vi "read data.vi"(8 "error in (no error)":errorcluster, 9 "pDMAStatus":i32[](array[numeric]), 10 "Buffer":u16[](array[numeric]), 11 "task":T1={"Task Info"={"Accele Task"=[], "Simulate"=FALSE, "采样率"={"AISampleRate"=10123, "CouplingType"=10000, "Butter"=1000}, "Trig"={"PreTrigCNT"=0, "TriggerMode"=enum."中间触发", "TriggerSource"=enum."软件触发", "ATRTriggerChannel"=enum."通道0", "TriggerDir"=enum."下降沿触发", "TrigLevelVolt"=0.0, "bAvailableTrig"=FALSE}, "clock"={"EN"=FALSE, "clocksource"=enum."内部时钟", "outclocksource"=enum."Trig0"}, "delay(S)"=0.0}, "datain"={"nSegmentCount"=0, "chaneldataSize"=8192, "t0 in"=timestamp(0 s since 1904-01-01), "nsegmentsize"=0, "chanelcouter"=0}, "times"=0.0, "timer"=[], "\nen"=FALSE} {"Task Info"."采样率"."CouplingType" items=["直流耦合", "交流耦合"]}) -> (0 "error out":errorcluster, 2 "Data":waveform(dbl)[](array[waveform]), 3 "task out":T1={"Task Info"={"Accele Task"=[], "Simulate"=FALSE, "采样率"={"AISampleRate"=10123, "CouplingType"=10000, "Butter"=1000}, "Trig"={"PreTrigCNT"=0, "TriggerMode"=enum."中间触发", "TriggerSource"=enum."软件触发", "ATRTriggerChannel"=enum."通道0", "TriggerDir"=enum."下降沿触发", "TrigLevelVolt"=0.0, "bAvailableTrig"=FALSE}, "clock"={"EN"=FALSE, "clocksource"=enum."内部时钟", "outclocksource"=enum."Trig0"}, "delay(S)"=0.0}, "datain"={"nSegmentCount"=0, "chaneldataSize"=8192, "t0 in"=timestamp(0 s since 1904-01-01), "nsegmentsize"=0, "chanelcouter"=0}, "times"=0.0, "timer"=[], "\nen"=FALSE} {"Task Info"."采样率"."CouplingType" items=["直流耦合", "交流耦合"]})   [LabVIEW 2009]
uses:
  <vilib>/Utility/TradDaqScaling.llb/Convert Thermocouple Reading (waveform).vi
  Data.vi
  PCI8532_32.dll
  Ctrls/Acceleration Channel Config_Ctrls-某型振动实验台测试系统.ctl
  Ctrls/Sample Information.ctl
  Ctrls/Trig.ctl
  Ctrls/clock.ctl
  Ctrls/Task Info.ctl
  Ctrls/task.ctl
  Ctrls/DATA info.ctl
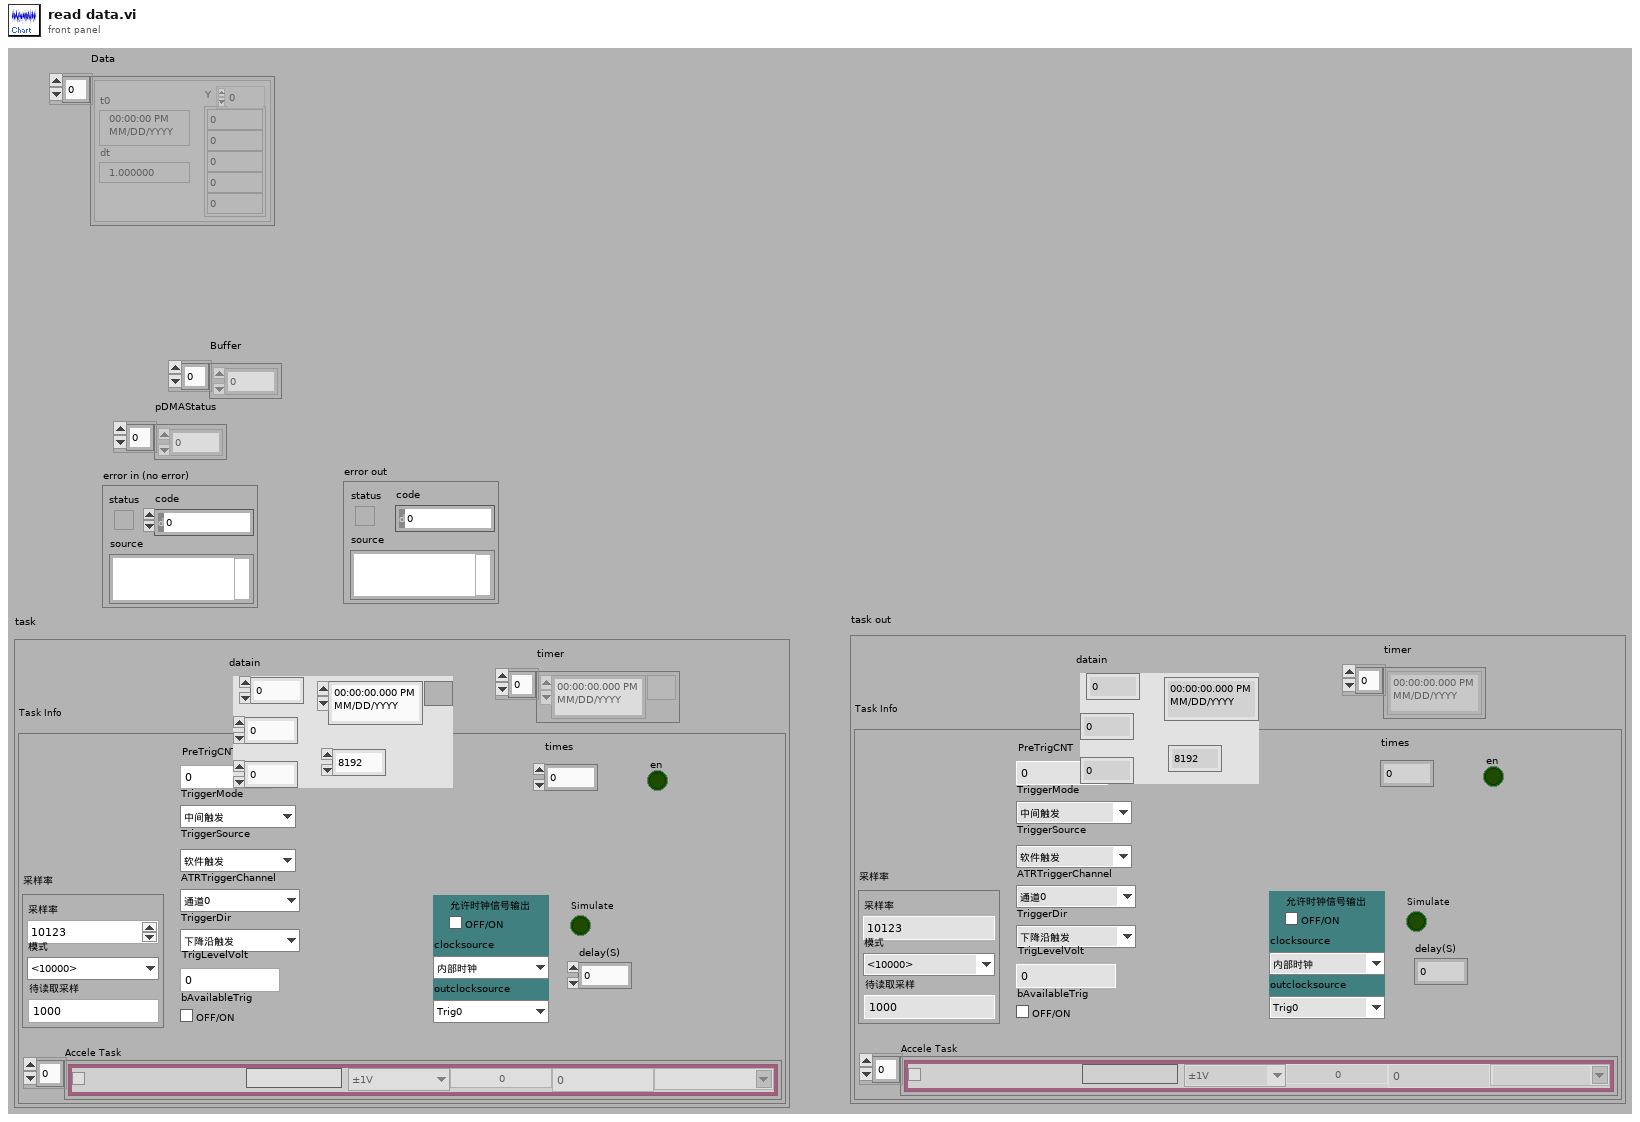
[diagram p1: front panel]
types:
  T1 = typedef "task.ctl" = cluster{"Task Info":T2, "datain":T7, "times":dbl, "timer":timestamp[], "\nen":bool}
  T2 = typedef "Task Info.ctl" = cluster{"Accele Task":T3[], "Simulate":bool, "采样率":T4, "Trig":T5, "clock":T6, "delay(S)":dbl}
  T3 = typedef "Acceleration Channel Config_Ctrls-某型振动实验台测试系统.ctl" = cluster{"Enable":bool, "Name":string, "range":enum16{"±1V", "±5V"}, "SensValue":dbl, "PhysicalName":string, "off":dbl, "Sensunits":string}
  T4 = typedef "Sample Information.ctl" = cluster{"AISampleRate":i32, "CouplingType":i32, "Butter":i32}
  T5 = typedef "Trig.ctl" = cluster{"PreTrigCNT":i32, "TriggerMode":enum16{"中间触发", "后触发", "预触发", "硬件延时触发"}, "TriggerSource":enum16{"软件触发", "DTR信号源", "ATR信号源", "Triger信号触发"}, "ATRTriggerChannel":enum16{"通道0", "通道1", "通道2", "通道3"}, "TriggerDir":enum16{"下降沿触发", "上升沿触发", "上下边没均触发"}, "TrigLevelVolt":sgl, "bAvailableTrig":bool}
  T6 = typedef "clock.ctl" = cluster{"EN":bool, "clocksource":enum16{"内部时钟", "外部时钟"}, "outclocksource":enum16{"Trig0", "Trig1", "Trig2", "Trig3", "Trig4", "Trig5", "Trig6", "Trig7", "PXI_STAR"}}
  T7 = typedef "DATA info.ctl" = cluster{"nSegmentCount":i32, "chaneldataSize":i32, "t0 in":timestamp, "nsegmentsize":i32, "chanelcouter":i32}
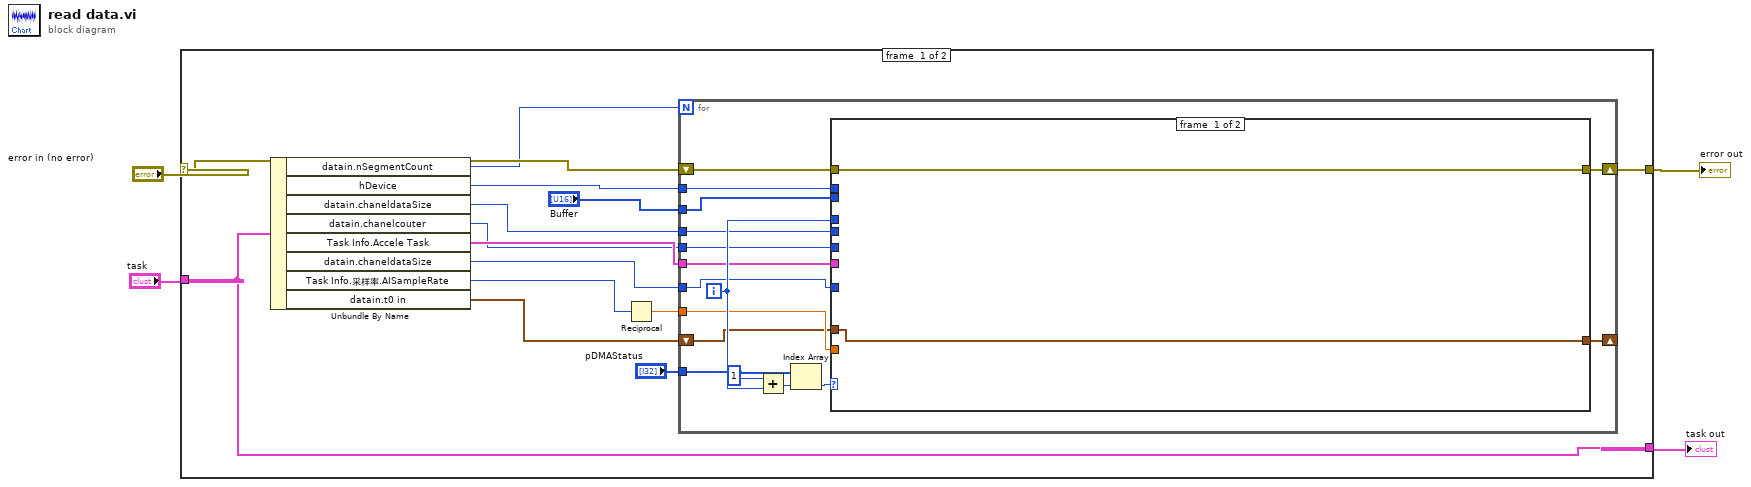
[diagram p0: block diagram]
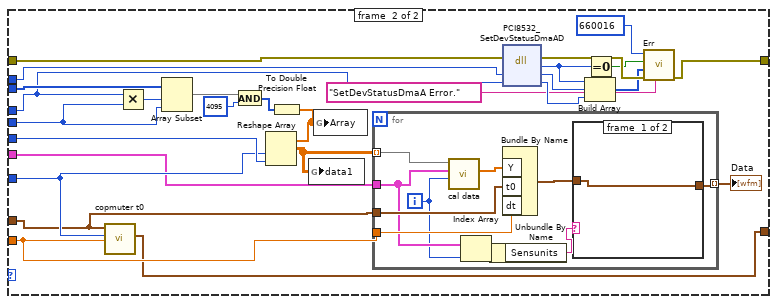
[diagram p2: hidden frame]
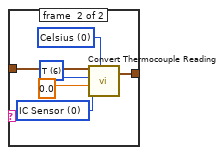
[diagram p3: hidden frame]
diagram:
  n1 = case shown="无错误" "error in (no error)" {
    selector: "error in (no error)" -> [w16 w81]
    tunnel: [w15 w81] -> w3
    tunnel: "task" -> [w13 w82]
    tunnel: [w13 w82] -> w1
    frame #0 {
      n2 = Unbundle By Name(w13) -> ("datain.nSegmentCount"=w12:i32, "hDevice"=w11:i32, "datain.chaneldataSize"=w10:i32, "datain.chanelcouter"=w5:i32, "Task Info.Accele Task"=w7:T3[], "datain.chaneldataSize"=w8:i32, "Task Info.采样率.AISampleRate"=w6:i32, "datain.t0 in"=w9:timestamp)
      n3 = Reciprocal(x=w6) -> (1/x=w14:dbl)
      n4 = for {
        N: w12 -> [_]
        tunnel: "pDMAStatus" -> [w34]
        tunnel: "Buffer" -> [w32]
        shift-right: [w27] -> w15
        shift-left: w16 -> [w28]
        tunnel: w11 -> [w26]
        tunnel: w7 -> [w25]
        tunnel: w14 -> [w24]
        tunnel: w8 -> [w22]
        tunnel: w10 -> [w21]
        tunnel: w5 -> [w20]
        shift-right: [w19] -> _
        shift-left: w9 -> [w23]
        i -> [w30]
        n5 = Add(x=1, y=w30) -> (x+y=w29:i32)
        n6 = Index Array(array=w34, index=w29) -> (element=w33:i32)
        n7 = case shown="1" w33 {
          tunnel: w30 -> [_ w53]
          tunnel: w32 -> [_ w63]
          tunnel: w28 -> [w36 w57]
          tunnel: [w36 w46] -> w27
          tunnel: w26 -> [_ w56]
          tunnel: w25 -> [_ w50]
          tunnel: w24 -> [_ w54]
          tunnel: w21 -> [_ w55]
          tunnel: w23 -> [w35 w49]
          tunnel: w22 -> [_ w51]
          tunnel: w20 -> [_ w52]
          tunnel: [w35 w48] -> w19
          frame #0 {
          }
          frame #1 {
            n8 = call "copmuter t0.vi"("time"=w54, "nchanelSize"=w51, "t0 in"=w49) -> ("t0 out"=w48:timestamp)  [unwired: 1 in, 7 out]
            n9 = Multiply(x=w53, y=w55) -> (x*y=w62:i32)
            n10 = Array Subset(array=w63, index=w62, length=w55) -> (w59:u16[])
            n11 = And(x=w59, y=4095) -> (x .and. y?=w60:i32[])
            n12 = To Double Precision Float(number=w60) -> (double precision float=w37:dbl[])
            n13 = Reshape Array(w37, w51, w52) -> (w38:dbl[][])
            n14 = global write "Data.vi" "data1"(w38) -> ()
            n15 = global write "Data.vi" "Array"(w37) -> ()
            n16 = for {
              tunnel: [w68] -> w58 mode=indexing
              tunnel: w54 -> [w73]
              tunnel: w49 -> [w70]
              tunnel: w38 -> [w72] mode=indexing
              tunnel: w50 -> [w67]
              i -> [w66]
              n17 = call "cal data.vi"("输入簇"=w66, "range"=w67, "data"=w72) -> ("data out"=w71:dbl[])  [unwired: 8 out]
              n18 = Index Array(array=w67, index=w66) -> (element=w65:T3)
              n19 = Unbundle By Name(w65) -> ("Sensunits"=w64:string)
              n20 = Bundle By Name("Y"=w71, "t0"=w70, "dt"=w73) -> (w69:waveform(dbl))  [unwired: 1 out]
              n21 = case shown="\"℃\"" w64 {
                tunnel: w69 -> [w74 w80]
                tunnel: [w74 w75] -> w68
                frame #0 {
                }
                frame #1 {
                  w76 = u16 0 items=["IC Sensor", "Thermistor"] ("CJC Sensor(0)")
                  w78 = u16 6 items=["B", "E", "J", "K", "R", "S", "T", "N"] ("ThermocoupleType")
                  w79 = u16 0 items=["Celsius", "Fahrenheit", "Kelvin", "Rankine"] ("Temperature Units (C)")
                  n22 = call-poly <vilib>:"Convert Thermocouple Reading.vi"("Temperature Units (C)"=w79, "CJC Sensor(0)"=w76, "CJC Voltage"=sgl 0.0, "ThermocoupleType"=w78, "Voltage Waveform"=w80) -> ("Temperature Waveform"=w75:waveform(dbl))  [unwired: 1 in, 1 out]
                }
              }
            }
            "Data" <- w58
            n23 = dll-call lib="PCI8532_32.dll" fn="PCI8532_SetDevStatusDmaAD" label="SetDevStatusDmaAD"(error in=w57, "hDevice"=w56, "iClrBufferID"=w53) -> (error out=w47:errorcluster, "返回类型"=w44:i32, "hDevice"=w43:i32, "iClrBufferID"=w42:i32)  [unwired: 2 in, 1 out]
            n24 = Build Array(w44, w43, w42) -> (w41:i32[])
            n25 = Equal To 0?(x=w44) -> (x = 0?=w45:bool)
            n26 = call "Err.vi"("source"="SetDevStatusDmaA Error.", "error in (no error)"=w47, "Par"=w41, "error?"=w45, "code"=660016) -> ("error out"=w46:errorcluster)  [unwired: 6 out]
          }
        }
      }
    }
    frame #1 {
    }
  }
  "error out" <- w3
  "task out" <- w1
